vi "Ready.vi"(0 "result_from_call in":refnum<class "result_from_call.lvclass">, 3 "error in (no error)":errorcluster) -> (7 "result_from_call out":refnum<class "result_from_call.lvclass">, 8 "ready":bool, 10 "error out":errorcluster)   [LabVIEW 2015, in "result_from_call.lvclass"]
uses:
  result_from_call.lvclass
  result_from_call.lvclass/result_from_call.ctl
  result.lvclass
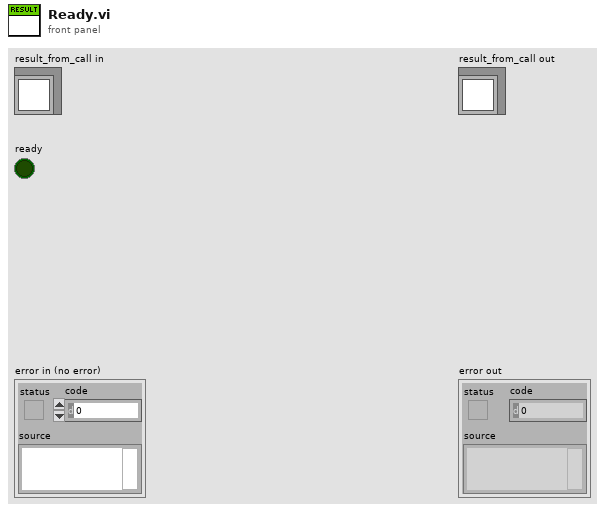
[diagram p1: front panel]
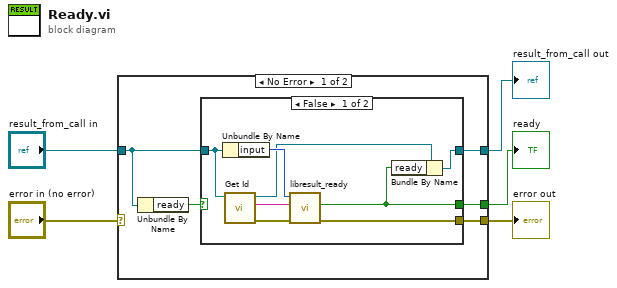
[diagram p0: block diagram]
diagram:
  n1 = case shown="No Error" "error in (no error)" {
    selector: "error in (no error)" -> [_ w21]
    tunnel: [w6 w21] -> w4
    tunnel: [w7 w22] -> w2
    tunnel: "result_from_call in" -> [w8 w22]
    tunnel: [w9 _] -> w1
    frame No Error {
      n2 = Unbundle By Name(w8) -> ("ready"=w10:bool)
      n3 = case shown="False" w10 {
        selector: w10 -> [_ w20]
        tunnel: [w17 w20] -> w9
        tunnel: w8 -> [w11 w19]
        tunnel: [w18 w19] -> w7
        tunnel: [w16 _] -> w6
        frame False {
          n4 = Unbundle By Name(w11) -> ("input"=w15:i32)
          n5 = call "Get Id.vi"("result in"=w11) -> ("error out"=w14:errorcluster, "id"=w13:string, "result out"=w12:refnum<class "result_from_call.lvclass">)  [unwired: 8 in]
          n6 = call "libresult_ready.vi"("error in (no error)"=w14, "id"=w13, "input"=w15) -> ("error out"=w16:errorcluster, "is"=w17:bool)  [unwired: 7 in]
          n7 = Bundle By Name(cluster=w12, "ready"=w17) -> (w18:refnum<class "result_from_call.lvclass">)
        }
        frame True {
        }
      }
    }
    frame Error {
    }
  }
  "error out" <- w4
  "result_from_call out" <- w2
  "ready" <- w1
